vi "LTS60_Serial_init.vi"(8 "err_in":errorcluster, 11 "mWADC_Port":refnum<visa-resource-name>) -> (0 "error out":errorcluster, 3 "reference out":refnum<visa-resource-name>)   [LabVIEW 2019]
uses:
  <vilib>/Instr/_visa.llb/VISA Flush IO Buffer Mask.ctl
panel:
  in  "Mask":T1=16 items=["Flush Receive Buffer"=16, "Write Transmit Buffer to Device"=32, "Flush Receive Buffer (No I/O)"=64, "Flush Transmit Buffer"=128]
  in  "Message Based Settings:Suppress End Enable":bool
  in  "Message Based Settings:Send End Enable":bool
  in  "Message Based Settings:Termination Character Enable":bool
  in  "Serial Settings:End Mode for Writes":u16(ring) items=["None", "Last Bit", "TermChar", "Break"]
  in  "Serial Settings:End Mode for Reads":u16(ring) items=["None", "Last Bit", "TermChar"]
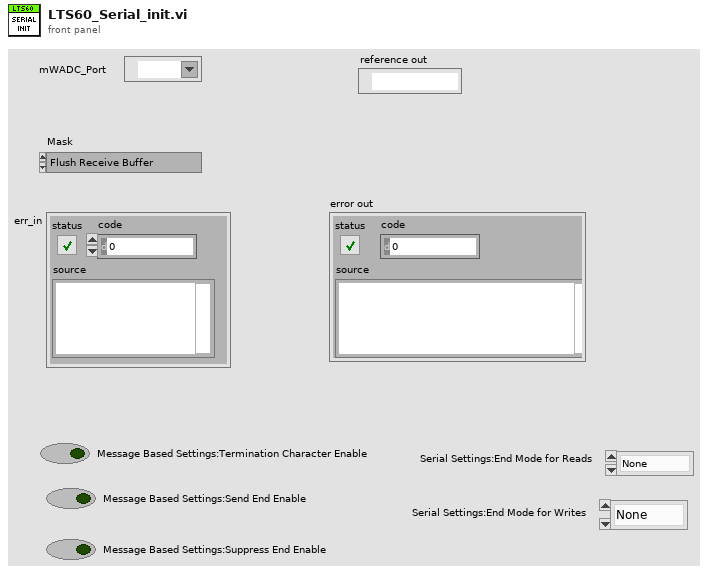
[diagram p1: front panel]
types:
  T1 = typedef "VISA Flush IO Buffer Mask.ctl" = u16
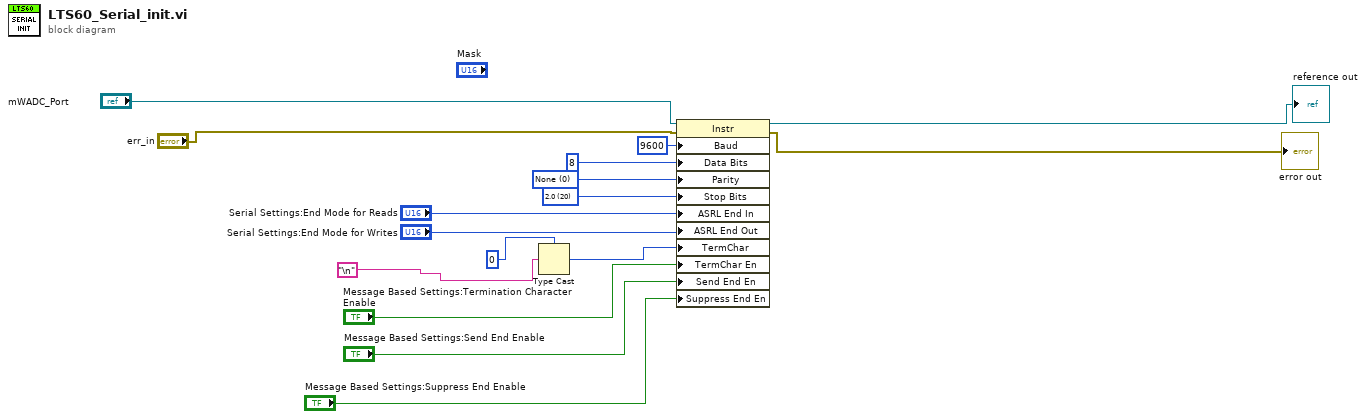
[diagram p0: block diagram]
diagram:
  w14 = u16 20 items=["1.0"=10, "1.5"=15, "2.0"=20] ("Serial Settings:Stop Bits")
  w15 = u16 0 items=["None", "Odd", "Even", "Mark", "Space"] ("Serial Settings:Parity")
  n1 = Type Cast(type=u8 0, x="\n") -> (*(type *) &x=w10:u8)
  n2 = property class="Instr"(reference="mWADC_Port", error in="err_in", "Baud"=u32 9600 ("Serial Settings:Baud Rate"), "Data Bits"=u16 8 ("Serial Settings:Data Bits"), "Parity"=w15, "Stop Bits"=w14, "ASRL End In"="Serial Settings:End Mode for Reads", "ASRL End Out"="Serial Settings:End Mode for Writes", "TermChar"=w10, "TermChar En"="Message Based Settings:Termination Character Enable", "Send End En"="Message Based Settings:Send End Enable", "Suppress End En"="Message Based Settings:Suppress End Enable") -> (reference out=→"reference out":refnum<visa-resource-name>, error out=→"error out":errorcluster)
